vi "Disconnect.vi"(8 "error in (no error)":errorcluster, 11 "Jiaxin_Stepper_Controller.lvlib:Jiaxin_Stepper.lvclass":refnum<class "Jiaxin_Stepper.lvclass">) -> (0 "error out":errorcluster, 3 "Jiaxin_Stepper_Controller.lvlib:Jiaxin_Stepper.lvclass":refnum<class "Jiaxin_Stepper.lvclass">)   [LabVIEW 2023, in "Jiaxin_Stepper_Controller.lvlib" / "Jiaxin_Stepper.lvclass"]
uses:
  Jiaxin_Stepper/Jiaxin_Stepper.lvclass
  Jiaxin_Stepper/Jiaxin_Stepper.lvclass/Jiaxin_Stepper.ctl
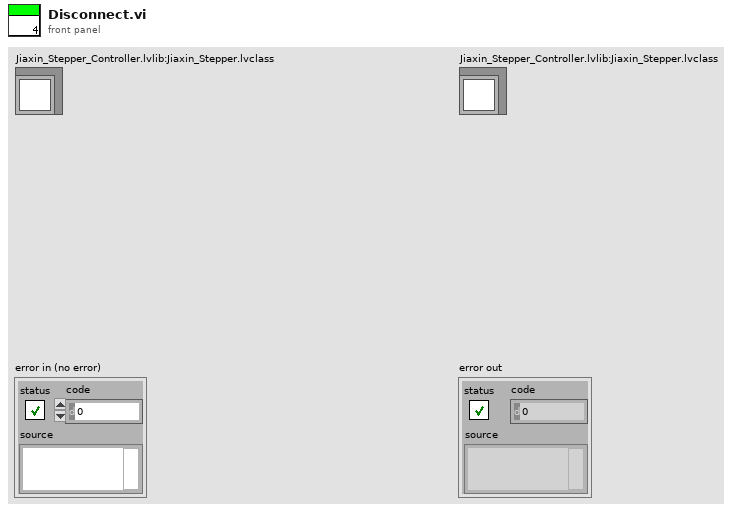
[diagram p1: front panel]
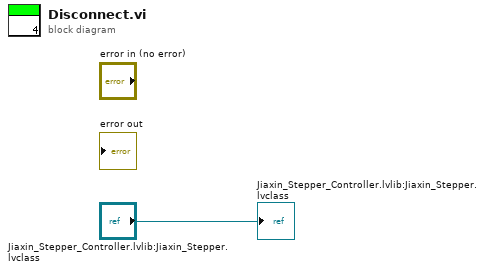
[diagram p0: block diagram]
diagram:
  "Jiaxin_Stepper_Controller.lvlib:Jiaxin_Stepper.lvclass" <- "Jiaxin_Stepper_Controller.lvlib:Jiaxin_Stepper.lvclass"
